vi "Read Float.vi"(8 "error in (no error)":errorcluster, 10 "Key":string, 11 "FlexWorktable in":refnum<class "FlexWorktable.lvclass">) -> (0 "error out":errorcluster, 2 "Float out":dbl, 3 "FlexWorktable out":refnum<class "FlexWorktable.lvclass">)   [LabVIEW 2017, in "FlexWorktable.lvclass"]
uses:
  FlexWorktable.lvclass
  FlexWorktable.lvclass/FlexWorktable.ctl
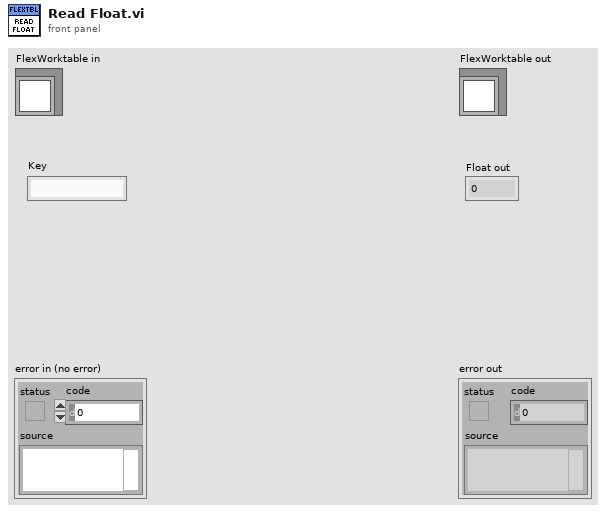
[diagram p1: front panel]
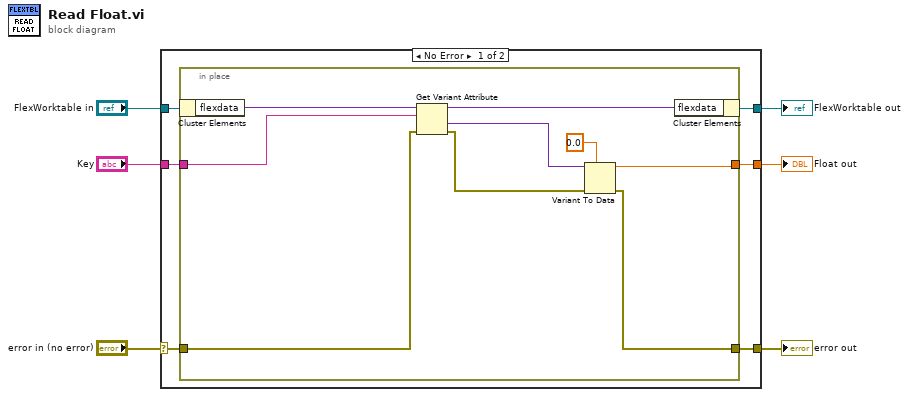
[diagram p0: block diagram]
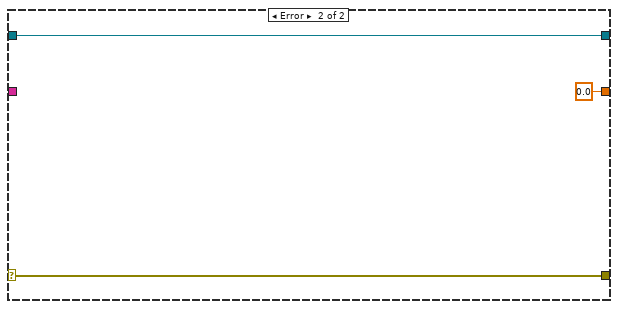
[diagram p2: hidden frame]
diagram:
  n1 = case shown="No Error" "error in (no error)" {
    selector: "error in (no error)" -> [w9 w24]
    tunnel: [w8 w24] -> w5
    tunnel: [w7 w23] -> w3
    tunnel: "FlexWorktable in" -> [w12 w23]
    tunnel: "Key" -> [w11 _]
    tunnel: [w10 0.0] -> w1
    frame No Error {
      n2 = in-place {
        in-place-border: w11 -> [w19]
        in-place-border: [w13] -> w10
        in-place-border: w9 -> [w18]
        in-place-border: [w14] -> w8
        n3 = in-place-cluster #1(w12) -> ("flexdata"=w21:variant)
        n4 = Get Variant Attribute(Variant=w21, name=w19, error in=w18) -> (duplicate Variant=w20:variant, value=w17:variant, error out=w15:errorcluster)  [unwired: 1 in, 1 out]
        n5 = Variant To Data(error in=w15, type=0.0, Variant=w17) -> (data=w13:dbl, error out=w14:errorcluster)
        n6 = in-place-cluster #1("flexdata"=w20) -> (w7:refnum<class "FlexWorktable.lvclass">)
      }
    }
    frame Error {
    }
  }
  "error out" <- w5
  "FlexWorktable out" <- w3
  "Float out" <- w1
